vi "Write.vi"(8 "error in (no error)":errorcluster, 10 "command":string, 11 "HAL in":refnum<class "HAL.lvclass">) -> (0 "error out":errorcluster, 3 "HAL out":refnum<class "HAL.lvclass">)   [LabVIEW 2019, in "Instrument.lvlib" / "HAL.lvclass"]
doc: "Override to <b>open</b> a connection to your instrument."
uses:
  HAL.lvclass
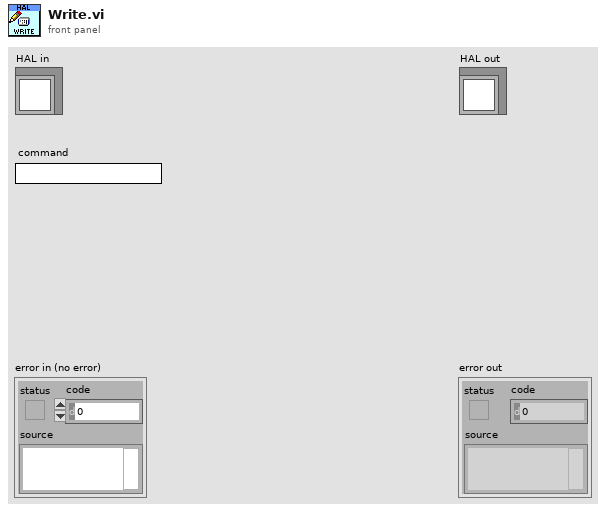
[diagram p1: front panel]
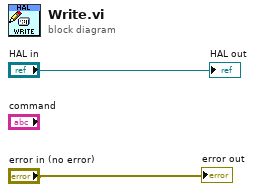
[diagram p0: block diagram]
diagram:
  "error out" <- "error in (no error)"
  "HAL out" <- "HAL in"
